vi "z_scan_read.vi"(11 "address in":u32) -> (1 "intensity":u16, 2 "z-value":i16, 3 "address out":u32)   [LabVIEW 2010]
uses:
  <vilib>/rvi/DataTransferAndStorage/Container/XNode/niFpgaContainer.xnode
  <vilib>/rvi/Memory/Memory_Emulation/nirvimemoryEmulationManagerCache_GetValue.vi
  <vilib>/rvi/DataTransferAndStorage/Container/Common/niFpgaContainerGetUniqueNameForEmu.vi
  <vilib>/rvi/Memory/Memory_Emulation/nirvimemoryEmulationManagerCache_InsertValue.vi
  <vilib>/Utility/error.llb/Clear Errors.vi
  <vilib>/rvi/Memory/Memory_Emulation/nirvimemoryEmulationManagerCache_SetValue.vi
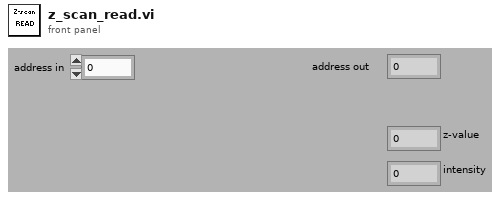
[diagram p1: front panel]
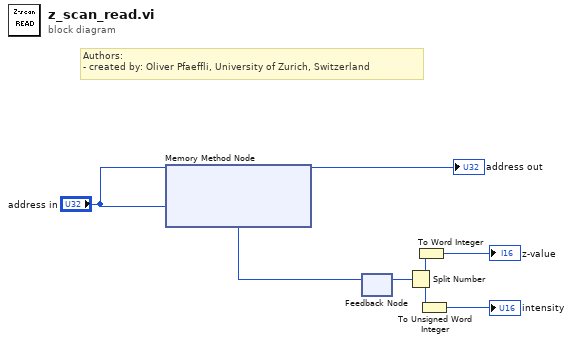
[diagram p0: block diagram]
diagram:
  # "Authors: \n- created by: Oliver Pfaeffli, University of Zurich, Switzerland"
  n1 = xnode ("Memory Method Node")("Address"="address in") -> ("Data"=w2:u32)  [unwired: 1 in, 1 out]
  n2 = feedback #1() -> (w1:u32)  [unwired: 1 in]
  n3 = feedback-in #1(w2) -> ()
  n4 = Split Number(x=w1) -> (hi(x)=w4:u16, lo(x)=w3:u16)
  n5 = To Word Integer(number=w4) -> (16bit integer=→"z-value":i16)
  n6 = To Unsigned Word Integer(number=w3) -> (unsigned 16bit integer=→"intensity":u16)
  "address out" <- "address in"
